vi "LSMcontroller_v66_improvedwfhandling.vi"() -> ()   [LabVIEW 2015] (continued)
                        n3642 = call "waveformsAObuffer.vi"("command"="get") -> ("AO wf out"=w516:waveform(dbl)[])  [unwired: 1 in]
                        n3643 = call "waveformsDObuffer.vi"("command"="get") -> ("DO wf out"=w513:digitalwaveform[])  [unwired: 1 in]
                        n3644 = Delete From Array(array=w516, length=1, index=w519) -> (array with subset deleted=w508:waveform(dbl)[])  [unwired: 1 out]
                        n3645 = call "correctwaveformsizetemp.vi"("new sampling frequency (Hz)"=w503, "start"=FALSE, "reference waveforms to"=w507, "Analog waveforms in"=w508, "stop"=FALSE, "Digital waveforms in"=w513) -> ("analog wf out"=w511:waveform(dbl)[], "Digital wf out"=w509:digitalwaveform[], "measpoints"=w505:i32)
                        n3646 = local write "Analog Lines Plot"(w511) -> ()
                        n3647 = call "GetNumCamFramesv2.vi"("Digital Waveform Graph"=w509) -> ("Numeric"=w510:i32)  [unwired: 10 in]
                        n3648 = local write "Digital Lines Plot"(w509) -> ()
                        n3649 = call "waveformsAObuffer.vi"("AO wf in"=w511, "command"="set") -> ()  [unwired: 1 out]
                        n3650 = call "waveformsDObuffer.vi"("DO wf in"=w509, "command"="set") -> ()  [unwired: 1 out]
                        n3651 = local read "wavdet"() -> (w506:bool)
                        n3652 = local write "Total Camera Frames"(w510) -> ()
                        n3653 = case shown="True" w506 {
                          tunnel: w505 -> [_ w522]
                          frame False {
                          }
                          frame True {
                            n3654 = local write "# of frames"(w522) -> ()
                          }
                        }
                      }
                    }
                  }
                  frame #6 {
                    w523 = FALSE ("remAO")
                    n3655 = local read "finite samples"() -> (w524:bool)
                    n3656 = local read "continuous"() -> (w525:bool)
                    n3657 = local read "wavdet"() -> (w526:bool)
                    n3658 = call "2pparameters.vi"("command"="get") -> ("params out"=w529:T10)  [unwired: 1 in]
                    n3659 = Bundle By Name(cluster=w529, "finite"=w524, "cont"=w525, "wavdet"=w526) -> (w527:T10)
                    n3660 = local write "remAO"(w523) -> ()
                    n3661 = property on="Rem AO wave" class="Bool (strict)"("Val(Sgnl)"=w523) -> ()  [unwired: 2 in, 2 out]
                    n3662 = call "2pparameters.vi"("Params in"=w527, "command"="set") -> ()  [unwired: 1 out]
                  }
                }
              }
            }
          }
          event "Add DO wave": Value Change {
            n3663 = event-data() -> ("NewVal"=w531:bool)  [unwired: 1 in, 5 out]
            n3664 = case shown="True" w531 {
              frame False {
              }
              frame True {
                n3665 = stacked-sequence {
                  seq-local: [_ _ _ _ _ w691 _ _] -> [_ _ _ _ _ _ w706 _]
                  frame #0 {
                    n3666 = local read "Measurement"() -> (w532:T4)
                    n3667 = case shown="\"X-Y-t movie\", Default" w532 {
                      frame "X-Y-t movie", Default {
                        n3668 = local read "avpp"() -> (w553:i32)
                        n3669 = local read "Angle ref"() -> (w552:dbl)
                        n3670 = local read "ROI Type"() -> (w551:u16)
                        n3671 = local read "xpixels ref"() -> (w548:i32)
                        n3672 = local read "Vx-min ref"() -> (w547:dbl)
                        n3673 = local read "Vx-max ref"() -> (w546:dbl)
                        n3674 = local read "ypixels ref"() -> (w544:i32)
                        n3675 = local read "Vy-min ref"() -> (w545:dbl)
                        n3676 = local read "Vy-max ref"() -> (w541:dbl)
                        n3677 = local read "Sampling rate"() -> (w535:dbl)
                        n3678 = local read "finite samples"() -> (w536:bool)
                        n3679 = local read "continuous"() -> (w539:bool)
                        n3680 = local read "wavdet"() -> (w540:bool)
                        n3681 = local read "# of frames"() -> (w538:i32)
                        n3682 = local read "maxbufferAI"() -> (w537:i32)
                        n3683 = local read "Override AI buffer"() -> (w533:bool)
                        n3684 = call "2pparameters.vi"("command"="get") -> ("params out"=w550:T10)  [unwired: 1 in]
                        n3685 = Bundle By Name(cluster=w550, "type"="X-Y-t movie", "avpp"=w553, "Angle Img"=w552, "Xpixels Img"=w548, "Vx-min Img"=w547, "VX-max Img"=w546, "Ypixels Img"=w544, "Vy-min Img"=w545, "Vy-max Img"=w541, "srate"=w535, "srate Img"=w535, "finite"=w536, "cont"=w539, "wavdet"=w540, "measpoints"=w538, "maxbufferAI"=w537, "Drawing Mode"=w551, "Vz-reset"=0.0, "AIoverride"=w533) -> (w542:T10)
                        n3686 = call "2pparameters.vi"("Params in"=w542, "command"="set") -> ()  [unwired: 1 out]
                      }
                      frame "X-Y-Z stack" {
                        n3687 = call "2pparameters.vi"("command"="get") -> ("params out"=w557:T10)  [unwired: 1 in]
                        n3688 = Bundle By Name(cluster=w557, "type"="X-Y-Z stack") -> (w555:T10)
                        n3689 = call "2pparameters.vi"("Params in"=w555, "command"="set") -> ()  [unwired: 1 out]
                      }
                      frame "Lifetime (scan)" {
                        n3690 = call "2pparameters.vi"("command"="get") -> ("params out"=w562:T10)  [unwired: 1 in]
                        n3691 = Bundle By Name(cluster=w562, "type"="Lifetime (scan)") -> (w560:T10)
                        n3692 = call "2pparameters.vi"("Params in"=w560, "command"="set") -> ()  [unwired: 1 out]
                      }
                      frame "Lifetime (contour)" {
                        n3693 = local read "Vy-min draw"() -> (w572:dbl)
                        n3694 = local read "Vy-max draw"() -> (w571:dbl)
                        n3695 = local read "Vx-min draw"() -> (w574:dbl)
                        n3696 = local read "Vx-max draw"() -> (w573:dbl)
                        n3697 = local read "xpixels ref"() -> (w570:i32)
                        n3698 = local read "ypixels ref"() -> (w569:i32)
                        n3699 = local read "ROI Type"() -> (w568:u16)
                        n3700 = local read "srateAODOtt"() -> (w579:dbl)
                        n3701 = local read "# of frames"() -> (w584:i32)
                        n3702 = local read "refreshtime"() -> (w576:dbl)
                        n3703 = local read "Pel"() -> (w567:dbl)
                        n3704 = local read "bin"() -> (w582:dbl)
                        n3705 = local read "Override AI buffer"() -> (w565:bool)
                        n3706 = local read "finite samples"() -> (w591:bool)
                        n3707 = local read "srateAODOtt"() -> (w578:dbl)
                        n3708 = local read "srateAODOtt"() -> (w585:dbl)
                        n3709 = local read "continuous"() -> (w590:bool)
                        n3710 = local read "Angle ref"() -> (w575:dbl)
                        n3711 = local read "wavdet"() -> (w592:bool)
                        n3712 = local read "Vx-ref"() -> (w587:dbl)
                        n3713 = local read "Vy-ref"() -> (w589:dbl)
                        n3714 = local read "avpp"() -> (w588:i32)
                        n3715 = call "tt_timeandsamples.vi"("bin"=w582, "refreshtime"=w576, "srateAODOtt"=w579, "tot#ofsamples"=w584) -> ("refreshrate"=w580:dbl, "refreshbuffer"=w581:i32, "timetracecycles"=w586:i32)  [unwired: 5 in]
                        n3716 = local read "bin"() -> (w583:dbl)
                        n3717 = call "2pparameters.vi"("command"="get") -> ("params out"=w595:T10)  [unwired: 1 in]
                        n3718 = Bundle By Name(cluster=w595, "Drawing Mode"=w568, "measpoints"=w584, "tt_cycles"=w586, "refreshbuffer"=w581, "refreshrate"=w580, "Vx-ref"=w587, "Vy-ref"=w589, "srate"=w578, "finite"=w591, "cont"=w590, "wavdet"=w592, "avpp"=w588, "srateAODO"=w585, "bufferAI"=w581, "bin"=w583, "Angle Img"=w575, "Vxminref"=w574, "Vxmaxref"=w573, "Vyminref"=w572, "Vymaxref"=w571, "Xpixels Img"=w570, "Ypixels Img"=w569, "Pel"=w567, "Vz-reset"=0.0, "AIoverride"=w565, "type"="Lifetime (contour)") -> (w593:T10)
                        n3719 = Reciprocal(x=w580) -> (1/x=w577:dbl)
                        n3720 = local write "refreshtime"(w577) -> ()
                        n3721 = call "2pparameters.vi"("Params in"=w593, "command"="set") -> ()  [unwired: 1 out]
                      }
                      frame "X-Y-Z-t movie" {
                      }
                      frame "linescan" {
                      }
                      frame "Timetrace" {
                        n3722 = local read "Vy-min draw"() -> (w605:dbl)
                        n3723 = local read "Vy-max draw"() -> (w604:dbl)
                        n3724 = local read "Vx-min draw"() -> (w607:dbl)
                        n3725 = local read "Vx-max draw"() -> (w606:dbl)
                        n3726 = local read "xpixels ref"() -> (w603:i32)
                        n3727 = local read "ypixels ref"() -> (w602:i32)
                        n3728 = local read "ROI Type"() -> (w601:u16)
                        n3729 = local read "srateAODOtt"() -> (w612:dbl)
                        n3730 = local read "# of frames"() -> (w617:i32)
                        n3731 = local read "refreshtime"() -> (w609:dbl)
                        n3732 = local read "Pel"() -> (w600:dbl)
                        n3733 = local read "bin"() -> (w615:dbl)
                        n3734 = local read "Override AI buffer"() -> (w598:bool)
                        n3735 = local read "finite samples"() -> (w624:bool)
                        n3736 = local read "srateAODOtt"() -> (w611:dbl)
                        n3737 = local read "srateAODOtt"() -> (w618:dbl)
                        n3738 = local read "continuous"() -> (w623:bool)
                        n3739 = local read "Angle ref"() -> (w608:dbl)
                        n3740 = local read "wavdet"() -> (w625:bool)
                        n3741 = local read "Vx-ref"() -> (w620:dbl)
                        n3742 = local read "Vy-ref"() -> (w622:dbl)
                        n3743 = local read "avpp"() -> (w621:i32)
                        n3744 = call "tt_timeandsamples.vi"("bin"=w615, "refreshtime"=w609, "srateAODOtt"=w612, "tot#ofsamples"=w617) -> ("refreshrate"=w613:dbl, "refreshbuffer"=w614:i32, "timetracecycles"=w619:i32)  [unwired: 5 in]
                        n3745 = local read "bin"() -> (w616:dbl)
                        n3746 = call "2pparameters.vi"("command"="get") -> ("params out"=w628:T10)  [unwired: 1 in]
                        n3747 = Bundle By Name(cluster=w628, "Drawing Mode"=w601, "measpoints"=w617, "tt_cycles"=w619, "refreshbuffer"=w614, "refreshrate"=w613, "Vx-ref"=w620, "Vy-ref"=w622, "srate"=w611, "finite"=w624, "cont"=w623, "wavdet"=w625, "avpp"=w621, "srateAODO"=w618, "bufferAI"=w614, "bin"=w616, "Angle Img"=w608, "Vxminref"=w607, "Vxmaxref"=w606, "Vyminref"=w605, "Vymaxref"=w604, "Xpixels Img"=w603, "Ypixels Img"=w602, "Pel"=w600, "Vz-reset"=0.0, "AIoverride"=w598, "type"="Timetrace") -> (w626:T10)
                        n3748 = Reciprocal(x=w613) -> (1/x=w610:dbl)
                        n3749 = local write "refreshtime"(w610) -> ()
                        n3750 = call "2pparameters.vi"("Params in"=w626, "command"="set") -> ()  [unwired: 1 out]
                      }
                      frame "Lifetime (point)" {
                      }
                    }
                  }
                  frame #1 {
                    w631 = FALSE ("wavdet")
                    n3751 = call "2pparameters.vi"("command"="get") -> ("params out"=w635:T10)  [unwired: 1 in]
                    n3752 = Bundle By Name(cluster=w635, "finite"=w631, "cont"=w631, "wavdet"=TRUE) -> (w632:T10)
                    n3753 = call "2pparameters.vi"("Params in"=w632, "command"="set") -> ()  [unwired: 1 out]
                  }
                  frame #2 {
                    n3754 = local read "DO channels"() -> (w642:u16)
                    n3755 = call "2pparameters.vi"("command"="get") -> ("params out"=w640:T10)  [unwired: 1 in]
                    n3756 = in-place {
                      in-place-border: w642 -> [w646]
                      in-place-border: [w643] -> w637
                      n3757 = in-place-cluster #51(w640) -> ("aDO"=w645:u32[])
                      n3758 = call "add channel to active arrayv2.vi"("line array in"=w645, "line to add"=w646) -> ("line array out"=w644:u32[], "addition"=w643:bool)  [unwired: 1 out]
                      n3759 = in-place-cluster #51("aDO"=w644) -> (w638:T10)
                    }
                    n3760 = local write "addDO"(w637) -> ()
                    n3761 = call "2pparameters.vi"("Params in"=w638, "command"="set") -> ()  [unwired: 1 out]
                  }
                  frame #3 {
                    n3762 = local read "addDO"() -> (w647:bool)
                    n3763 = case shown="True" w647 {
                      frame False {
                      }
                      frame True {
                        n3764 = call "Used AO lines.vi"() -> ("used AO names"=w651:string[], "used AO lines"=w653:tag[])  [unwired: 2 in]
                        n3765 = control-ref of="Analog Lines Plot"() -> (w652:refnum<vi>)
                        n3766 = control-ref of="Digital Lines Plot"() -> (w650:refnum<vi>)
                        n3767 = call "Used DO lines.vi"() -> ("used DO names"=w649:string[], "used DO lines"=w648:tag[])  [unwired: 2 in]
                        n3768 = local write "Analog Used Lines"(w653) -> ()
                        n3769 = local write "Analog Used Names"(w651) -> ()
                        n3770 = local write "Digital Used Lines"(w648) -> ()
                        n3771 = local write "Digital Used Names"(w649) -> ()
                        n3772 = call "prepDOWaveplot.vi"("DigitalGraph in"=w650, "used DO names"=w649) -> ()  [unwired: 1 in]
                        n3773 = call "prepAOWaveplot.vi"("WaveformGraph in"=w652, "Analog Used Names"=w651) -> ()  [unwired: 1 in]
                      }
                    }
                  }
                  frame #4 {
                    n3774 = local read "addDO"() -> (w654:bool)
                    n3775 = case shown="True" w654 {
                      frame False {
                      }
                      frame True {
                        n3776 = local read "Build digital waveform tabs"() -> (w655:enum32{"Simple", "Matlab"})
                        n3777 = case shown="\"Matlab\"" w655 {
                          frame "Simple", Default {
                            n3778 = local read "Meastab"() -> (w657:enum32{"X-Y Image", "Linescan", "Timetrace"})
                            n3779 = call "waveformparamsv2.vi"("command"="get") -> ("Params out"=w671:T14)  [unwired: 4 in, 2 out]
                            n3780 = case shown="\"Timetrace\"" w657 {
                              tunnel: [w673 w674] -> w656
                              frame "X-Y Image", Default {
                                n3781 = local read "Sampling rate"() -> (w673:dbl)
                              }
                              frame "Timetrace" {
                                n3782 = local read "srateAODOtt"() -> (w674:dbl)
                              }
                            }
                            n3783 = Unbundle By Name(w671) -> ("DO parameters"=w669:T17)
                            n3784 = local read "Digital padding value"() -> (w660:dbl)
                            n3785 = local read "Digital time offset (s)"() -> (w661:dbl)
                            n3786 = local read "Digital phase (s)"() -> (w663:dbl)
                            n3787 = local read "Digital Freq (Hz)"() -> (w662:dbl)
                            n3788 = local read "Digital DC (%)"() -> (w664:dbl)
                            n3789 = Index Array(array=w669, index=0) -> (element=w668:T18)
                            n3790 = Bundle By Name(cluster=w668, "Digital DC (%)"=w664, "Digital phase"=w663, "Digital Freq (Hz)"=w662, "Sampling frequency (Hz)"=w656, "Digital time offset (s)"=w661, "padding value"=w660, "matlab wave file"=path "", "DOtab"=0.0) -> (w666:T18)
                            n3791 = Build Array(w666) -> (w665:T17)
                            n3792 = call "waveformparamsv2.vi"("command"="add DO", "add DO"=w665) -> ()  [unwired: 3 in, 3 out]
                          }
                          frame "Matlab" {
                            w678 = 0.0 ("DOtab")
                            n3793 = local read "Meastab"() -> (w676:enum32{"X-Y Image", "Linescan", "Timetrace"})
                            n3794 = call "waveformparamsv2.vi"("command"="get") -> ("Params out"=w687:T14)  [unwired: 4 in, 2 out]
                            n3795 = case shown="\"Timetrace\"" w676 {
                              tunnel: [w689 w690] -> w675
                              frame "X-Y Image", Default {
                                n3796 = local read "Sampling rate"() -> (w689:dbl)
                              }
                              frame "Timetrace" {
                                n3797 = local read "srateAODOtt"() -> (w690:dbl)
                              }
                            }
                            n3798 = Unbundle By Name(w687) -> ("DO parameters"=w685:T17)
                            n3799 = local read "Matlab waveform path DO"() -> (w677:path)
                            n3800 = local read "Matlab padding value DO"() -> (w680:dbl)
                            n3801 = Index Array(array=w685, index=0) -> (element=w684:T18)
                            n3802 = Bundle By Name(cluster=w684, "Digital DC (%)"=w678, "Digital phase"=w678, "Digital Freq (Hz)"=w678, "Sampling frequency (Hz)"=w675, "Digital time offset (s)"=w678, "padding value"=w680, "matlab wave file"=w677, "DOtab"=1.0) -> (w682:T18)
                            n3803 = Build Array(w682) -> (w681:T17)
                            n3804 = call "waveformparamsv2.vi"("command"="add DO", "add DO"=w681) -> ()  [unwired: 3 in, 3 out]
                          }
                        }
                      }
                    }
                  }
                  frame #5 {
                    n3805 = local read "addDO"() -> (w692:bool)
                    n3806 = case shown="True" w692 {
                      tunnel: [_ w693] -> w691
                      frame False {
                      }
                      frame True {
                        n3807 = property on="refwf" class="Ring (strict)"() -> ("RingText.Text"=w698:string)  [unwired: 2 in, 2 out]
                        n3808 = call "waveformsDObuffer.vi"("command"="get") -> ("DO wf out"=w697:digitalwaveform[])  [unwired: 1 in]
                        n3809 = call "waveformsAObuffer.vi"("command"="get") -> ("AO wf out"=w695:waveform(dbl)[])  [unwired: 1 in]
                        n3810 = call "referfencesize.vi"("Digital waveforms in"=w697, "Analog waveforms in"=w695, "reference waveforms to"=w698) -> ("number of samples"=w693:i32)  [unwired: 2 in]
                      }
                    }
                  }
                  frame #6 {
                    n3811 = local read "Build digital waveform tabs"() -> (w709:enum32{"Simple", "Matlab"})
                    n3812 = call "waveformparamsv2.vi"("command"="get last DO") -> ("last DO"=w708:T18)  [unwired: 4 in, 2 out]
                    n3813 = local read "Meastab"() -> (w702:enum32{"X-Y Image", "Linescan", "Timetrace"})
                    n3814 = call "waveformsDObuffer.vi"("command"="get") -> ("DO wf out"=w707:digitalwaveform[])  [unwired: 1 in]
                    n3815 = case shown="\"Simple\", Default" w709 {
                      tunnel: w708 -> [w726 w728]
                      tunnel: w706 -> [w725 _]
                      tunnel: [w724 w727] -> w705
                      frame "Simple", Default {
                        n3816 = call "simple digital from wf params.vi"("waveform params"=w726, "number of samples"=w725) -> ("digital waveform"=w724:digitalwaveform)
                      }
                      frame "Matlab" {
                        n3817 = call "matlabDOwffromparam.vi"("waveform params"=w728) -> ("digital waveform"=w727:digitalwaveform)
                      }
                    }
                    n3818 = property on="refwf" class="Ring (strict)"() -> ("RingText.Text"=w712:string)  [unwired: 2 in, 2 out]
                    n3819 = case shown="\"Timetrace\"" w702 {
                      tunnel: [w721 w722] -> w701
                      frame "X-Y Image", Default {
                        n3820 = local read "Sampling rate"() -> (w721:dbl)
                      }
                      frame "Timetrace" {
                        n3821 = local read "srateAODOtt"() -> (w722:dbl)
                      }
                    }
                    n3822 = call "waveformsAObuffer.vi"("command"="get") -> ("AO wf out"=w720:waveform(dbl)[])  [unwired: 1 in]
                    n3823 = Build Array (concatenate)(w707, w705) -> (w711:digitalwaveform[])
                    n3824 = call "correctwaveformsizetemp.vi"("new sampling frequency (Hz)"=w701, "start"=FALSE, "reference waveforms to"=w712, "Analog waveforms in"=w720, "stop"=FALSE, "Digital waveforms in"=w711) -> ("analog wf out"=w715:waveform(dbl)[], "Digital wf out"=w713:digitalwaveform[], "measpoints"=w703:i32)
                    n3825 = local write "Analog Lines Plot"(w715) -> ()
                    n3826 = call "GetNumCamFramesv2.vi"("Digital Waveform Graph"=w713) -> ("Numeric"=w714:i32)  [unwired: 10 in]
                    n3827 = local write "Digital Lines Plot"(w713) -> ()
                    n3828 = call "waveformsAObuffer.vi"("AO wf in"=w715, "command"="set") -> ()  [unwired: 1 out]
                    n3829 = call "waveformsDObuffer.vi"("DO wf in"=w713, "command"="set") -> ()  [unwired: 1 out]
                    n3830 = local write "Total Camera Frames"(w714) -> ()
                    n3831 = local read "wavdet"() -> (w704:bool)
                    n3832 = case shown="True" w704 {
                      tunnel: w703 -> [_ w723]
                      frame False {
                      }
                      frame True {
                        n3833 = local write "# of frames"(w723) -> ()
                      }
                    }
                  }
                  frame #7 {
                    w730 = FALSE ("addAO")
                    n3834 = local read "Build digital waveform tabs"() -> (w729:enum32{"Simple", "Matlab"})
                    n3835 = case shown="\"Simple\", Default" w729 {
                      frame "Simple", Default {
                        n3836 = local write "not loadedDO"(FALSE ("not loadedDO")) -> ()
                      }
                      frame "Matlab" {
                        n3837 = local write "not loadedDOml"(FALSE ("not loadedDO")) -> ()
                      }
                    }
                    n3838 = local read "finite samples"() -> (w731:bool)
                    n3839 = local read "continuous"() -> (w732:bool)
                    n3840 = local read "wavdet"() -> (w733:bool)
                    n3841 = call "2pparameters.vi"("command"="get") -> ("params out"=w736:T10)  [unwired: 1 in]
                    n3842 = Bundle By Name(cluster=w736, "finite"=w731, "cont"=w732, "wavdet"=w733) -> (w734:T10)
                    n3843 = call "2pparameters.vi"("Params in"=w734, "command"="set") -> ()  [unwired: 1 out]
                    n3844 = local write "addDO"(w730) -> ()
                    n3845 = property on="Add DO wave" class="Bool (strict)"("Val(Sgnl)"=w730) -> ()  [unwired: 2 in, 2 out]
                  }
                }
              }
            }
          }
          event "DO channels": Value Change {
            n3846 = event-data() -> ()  [unwired: 1 in, 6 out]
            n3847 = local read "DO channels"() -> (w742:u16)
            n3848 = call "2pparameters.vi"("command"="get") -> ("params out"=w744:T10)  [unwired: 1 in]
            n3849 = Unbundle By Name(w744) -> ("aDO"=w743:u32[])
            n3850 = Search 1D Array(1D array=w743, element=w742) -> (index of element=w741:i32)  [unwired: 1 in]
            n3851 = Equal?(x=w741, y=-1.0) -> (x = y?=w740:bool)
            n3852 = case shown="False" w740 {
              tunnel: w741 -> [w759 _]
              frame False {
                n3853 = call "waveformparamsv2.vi"("command"="get") -> ("Params out"=w754:T14)  [unwired: 4 in, 2 out]
                n3854 = Unbundle By Name(w754) -> ("DO parameters"=w752:T17)
                n3855 = Index Array(array=w752, index=w759) -> (element=w758:T18)
                n3856 = Unbundle By Name(w758) -> ("Digital DC (%)"=w757:dbl, "Digital phase"=w756:dbl, "Digital Freq (Hz)"=w755:dbl, "Sampling frequency (Hz)"=w747:dbl, "Digital time offset (s)"=w751:dbl, "padding value"=w750:dbl, "matlab wave file"=w749:path, "DOtab"=w748:dbl)
                n3857 = local write "Build digital waveform tabs"(w748) -> ()
                n3858 = local write "Digital DC (%)"(w757) -> ()
                n3859 = local write "Matlab waveform path DO"(w749) -> ()
                n3860 = local write "Digital time offset (s)"(w751) -> ()
                n3861 = local write "Matlab padding value DO"(w750) -> ()
                n3862 = local write "Digital padding value"(w750) -> ()
                n3863 = local write "Sampling rate \ncurrent wf"(w747) -> ()
                n3864 = local write "Digital Freq (Hz)"(w755) -> ()
                n3865 = local write "Digital phase (s)"(w756) -> ()
              }
              frame True {
              }
            }
          }
          event "Rem DO wave": Value Change {
            n3866 = event-data() -> ("NewVal"=w760:bool)  [unwired: 1 in, 5 out]
            n3867 = case shown="True" w760 {
              frame False {
              }
              frame True {
                n3868 = stacked-sequence {
                  seq-local: [_ _ w866 _ _ _ _] -> [_ _ _ _ w885 w896 _]
                  frame #0 {
                    n3869 = local read "Measurement"() -> (w761:T4)
                    n3870 = case shown="\"linescan\"" w761 {
                      frame "X-Y-t movie", Default {
                        n3871 = local read "avpp"() -> (w782:i32)
                        n3872 = local read "Angle ref"() -> (w781:dbl)
                        n3873 = local read "ROI Type"() -> (w780:u16)
                        n3874 = local read "xpixels ref"() -> (w777:i32)
                        n3875 = local read "Vx-min ref"() -> (w776:dbl)
                        n3876 = local read "Vx-max ref"() -> (w775:dbl)
                        n3877 = local read "ypixels ref"() -> (w773:i32)
                        n3878 = local read "Vy-min ref"() -> (w774:dbl)
                        n3879 = local read "Vy-max ref"() -> (w770:dbl)
                        n3880 = local read "Sampling rate"() -> (w764:dbl)
                        n3881 = local read "finite samples"() -> (w765:bool)
                        n3882 = local read "continuous"() -> (w768:bool)
                        n3883 = local read "wavdet"() -> (w769:bool)
                        n3884 = local read "# of frames"() -> (w767:i32)
                        n3885 = local read "maxbufferAI"() -> (w766:i32)
                        n3886 = local read "Override AI buffer"() -> (w762:bool)
                        n3887 = call "2pparameters.vi"("command"="get") -> ("params out"=w779:T10)  [unwired: 1 in]
                        n3888 = Bundle By Name(cluster=w779, "type"="X-Y-t movie", "avpp"=w782, "Angle Img"=w781, "Xpixels Img"=w777, "Vx-min Img"=w776, "VX-max Img"=w775, "Ypixels Img"=w773, "Vy-min Img"=w774, "Vy-max Img"=w770, "srate"=w764, "srate Img"=w764, "finite"=w765, "cont"=w768, "wavdet"=w769, "measpoints"=w767, "maxbufferAI"=w766, "Drawing Mode"=w780, "Vz-reset"=0.0, "AIoverride"=w762) -> (w771:T10)
                        n3889 = call "2pparameters.vi"("Params in"=w771, "command"="set") -> ()  [unwired: 1 out]
                      }
                      frame "X-Y-Z stack" {
                        n3890 = call "2pparameters.vi"("command"="get") -> ("params out"=w786:T10)  [unwired: 1 in]
                        n3891 = Bundle By Name(cluster=w786, "type"="X-Y-Z stack") -> (w784:T10)
                        n3892 = call "2pparameters.vi"("Params in"=w784, "command"="set") -> ()  [unwired: 1 out]
                      }
                      frame "Lifetime (scan)" {
                        n3893 = call "2pparameters.vi"("command"="get") -> ("params out"=w791:T10)  [unwired: 1 in]
                        n3894 = Bundle By Name(cluster=w791, "type"="Lifetime (scan)") -> (w789:T10)
                        n3895 = call "2pparameters.vi"("Params in"=w789, "command"="set") -> ()  [unwired: 1 out]
                      }
                      frame "Lifetime (contour)" {
                        n3896 = local read "Vy-min draw"() -> (w801:dbl)
                        n3897 = local read "Vy-max draw"() -> (w800:dbl)
                        n3898 = local read "Vx-min draw"() -> (w803:dbl)
                        n3899 = local read "Vx-max draw"() -> (w802:dbl)
                        n3900 = local read "xpixels ref"() -> (w799:i32)
                        n3901 = local read "ypixels ref"() -> (w798:i32)
                        n3902 = local read "ROI Type"() -> (w797:u16)
                        n3903 = local read "srateAODOtt"() -> (w808:dbl)
                        n3904 = local read "# of frames"() -> (w813:i32)
                        n3905 = local read "refreshtime"() -> (w805:dbl)
                        n3906 = local read "Pel"() -> (w796:dbl)
                        n3907 = local read "bin"() -> (w811:dbl)
                        n3908 = local read "Override AI buffer"() -> (w794:bool)
                        n3909 = local read "finite samples"() -> (w820:bool)
                        n3910 = local read "srateAODOtt"() -> (w807:dbl)
                        n3911 = local read "srateAODOtt"() -> (w814:dbl)
                        n3912 = local read "continuous"() -> (w819:bool)
                        n3913 = local read "Angle ref"() -> (w804:dbl)
                        n3914 = local read "wavdet"() -> (w821:bool)
                        n3915 = local read "Vx-ref"() -> (w816:dbl)
                        n3916 = local read "Vy-ref"() -> (w818:dbl)
                        n3917 = local read "avpp"() -> (w817:i32)
                        n3918 = call "tt_timeandsamples.vi"("bin"=w811, "refreshtime"=w805, "srateAODOtt"=w808, "tot#ofsamples"=w813) -> ("refreshrate"=w809:dbl, "refreshbuffer"=w810:i32, "timetracecycles"=w815:i32)  [unwired: 5 in]
                        n3919 = local read "bin"() -> (w812:dbl)
                        n3920 = call "2pparameters.vi"("command"="get") -> ("params out"=w824:T10)  [unwired: 1 in]
                        n3921 = Bundle By Name(cluster=w824, "Drawing Mode"=w797, "measpoints"=w813, "tt_cycles"=w815, "refreshbuffer"=w810, "refreshrate"=w809, "Vx-ref"=w816, "Vy-ref"=w818, "srate"=w807, "finite"=w820, "cont"=w819, "wavdet"=w821, "avpp"=w817, "srateAODO"=w814, "bufferAI"=w810, "bin"=w812, "Angle Img"=w804, "Vxminref"=w803, "Vxmaxref"=w802, "Vyminref"=w801, "Vymaxref"=w800, "Xpixels Img"=w799, "Ypixels Img"=w798, "Pel"=w796, "Vz-reset"=0.0, "AIoverride"=w794, "type"="Lifetime (contour)") -> (w822:T10)
                        n3922 = Reciprocal(x=w809) -> (1/x=w806:dbl)
                        n3923 = local write "refreshtime"(w806) -> ()
                        n3924 = call "2pparameters.vi"("Params in"=w822, "command"="set") -> ()  [unwired: 1 out]
                      }
                      frame "X-Y-Z-t movie" {
                      }
                      frame "linescan" {
                      }
                      frame "Timetrace" {
                        n3925 = local read "Vy-min draw"() -> (w834:dbl)
                        n3926 = local read "Vy-max draw"() -> (w833:dbl)
                        n3927 = local read "Vx-min draw"() -> (w836:dbl)
                        n3928 = local read "Vx-max draw"() -> (w835:dbl)
                        n3929 = local read "xpixels ref"() -> (w832:i32)
                        n3930 = local read "ypixels ref"() -> (w831:i32)
                        n3931 = local read "ROI Type"() -> (w830:u16)
                        n3932 = local read "srateAODOtt"() -> (w841:dbl)
                        n3933 = local read "# of frames"() -> (w846:i32)
                        n3934 = local read "refreshtime"() -> (w838:dbl)
                        n3935 = local read "Pel"() -> (w829:dbl)
                        n3936 = local read "bin"() -> (w844:dbl)
                        n3937 = local read "Override AI buffer"() -> (w827:bool)
                        n3938 = local read "finite samples"() -> (w853:bool)
                        n3939 = local read "srateAODOtt"() -> (w840:dbl)
                        n3940 = local read "srateAODOtt"() -> (w847:dbl)
                        n3941 = local read "continuous"() -> (w852:bool)
                        n3942 = local read "Angle ref"() -> (w837:dbl)
                        n3943 = local read "wavdet"() -> (w854:bool)
                        n3944 = local read "Vx-ref"() -> (w849:dbl)
                        n3945 = local read "Vy-ref"() -> (w851:dbl)
                        n3946 = local read "avpp"() -> (w850:i32)
                        n3947 = call "tt_timeandsamples.vi"("bin"=w844, "refreshtime"=w838, "srateAODOtt"=w841, "tot#ofsamples"=w846) -> ("refreshrate"=w842:dbl, "refreshbuffer"=w843:i32, "timetracecycles"=w848:i32)  [unwired: 5 in]
                        n3948 = local read "bin"() -> (w845:dbl)
                        n3949 = call "2pparameters.vi"("command"="get") -> ("params out"=w857:T10)  [unwired: 1 in]
                        n3950 = Bundle By Name(cluster=w857, "Drawing Mode"=w830, "measpoints"=w846, "tt_cycles"=w848, "refreshbuffer"=w843, "refreshrate"=w842, "Vx-ref"=w849, "Vy-ref"=w851, "srate"=w840, "finite"=w853, "cont"=w852, "wavdet"=w854, "avpp"=w850, "srateAODO"=w847, "bufferAI"=w843, "bin"=w845, "Angle Img"=w837, "Vxminref"=w836, "Vxmaxref"=w835, "Vyminref"=w834, "Vymaxref"=w833, "Xpixels Img"=w832, "Ypixels Img"=w831, "Pel"=w829, "Vz-reset"=0.0, "AIoverride"=w827, "type"="Timetrace") -> (w855:T10)
                        n3951 = Reciprocal(x=w842) -> (1/x=w839:dbl)
                        n3952 = local write "refreshtime"(w839) -> ()
                        n3953 = call "2pparameters.vi"("Params in"=w855, "command"="set") -> ()  [unwired: 1 out]
                      }
                      frame "Lifetime (point)" {
                      }
                    }
                  }
                  frame #1 {
                    w860 = FALSE ("wavdet")
                    n3954 = call "2pparameters.vi"("command"="get") -> ("params out"=w864:T10)  [unwired: 1 in]
                    n3955 = Bundle By Name(cluster=w864, "finite"=w860, "cont"=w860, "wavdet"=TRUE) -> (w861:T10)
                    n3956 = call "2pparameters.vi"("Params in"=w861, "command"="set") -> ()  [unwired: 1 out]
                  }
                  frame #2 {
                    n3957 = local read "DO channels"() -> (w872:u16)
                    n3958 = call "2pparameters.vi"("command"="get") -> ("params out"=w870:T10)  [unwired: 1 in]
                    n3959 = in-place {
                      in-place-border: w872 -> [w877]
                      in-place-border: [w874] -> w867
                      in-place-border: [w873] -> w866
                      n3960 = in-place-cluster #52(w870) -> ("aDO"=w876:u32[])
                      n3961 = call "remove channel from active arrayv2.vi"("line array in"=w876, "line to remove"=w877) -> ("line array out"=w875:u32[], "removal"=w874:bool, "index"=w873:i32)
                      n3962 = in-place-cluster #52("aDO"=w875) -> (w868:T10)
                    }
                    n3963 = local write "remDO"(w867) -> ()
                    n3964 = call "2pparameters.vi"("Params in"=w868, "command"="set") -> ()  [unwired: 1 out]
                  }
                  frame #3 {
                    n3965 = local read "remDO"() -> (w878:bool)
                    n3966 = case shown="True" w878 {
                      frame False {
                      }
                      frame True {
                        n3967 = call "Used AO lines.vi"() -> ("used AO names"=w882:string[], "used AO lines"=w884:tag[])  [unwired: 2 in]
                        n3968 = local write "Analog Used Lines"(w884) -> ()
                        n3969 = local write "Analog Used Names"(w882) -> ()
                        n3970 = call "Used DO lines.vi"() -> ("used DO names"=w880:string[], "used DO lines"=w879:tag[])  [unwired: 2 in]
                        n3971 = control-ref of="Analog Lines Plot"() -> (w883:refnum<vi>)
                        n3972 = control-ref of="Digital Lines Plot"() -> (w881:refnum<vi>)
                        n3973 = local write "Digital Used Lines"(w879) -> ()
                        n3974 = local write "Digital Used Names"(w880) -> ()
                        n3975 = call "prepAOWaveplot.vi"("WaveformGraph in"=w883, "Analog Used Names"=w882) -> ()  [unwired: 1 in]
                        n3976 = call "prepDOWaveplot.vi"("DigitalGraph in"=w881, "used DO names"=w880) -> ()  [unwired: 1 in]
                      }
                    }
                  }
                  frame #4 {
                    n3977 = local read "remDO"() -> (w886:bool)
                    n3978 = case shown="True" w886 {
                      tunnel: w885 -> [_ w887]
                      frame False {
                      }
                      frame True {
                        n3979 = call "waveformparamsv2.vi"("command"="rem DO", "index"=w887) -> ()  [unwired: 3 in, 3 out]
                      }
                    }
                  }
                  frame #5 {
                    n3980 = local read "Meastab"() -> (w892:enum32{"X-Y Image", "Linescan", "Timetrace"})
                    n3981 = property on="refwf" class="Ring (strict)"() -> ("RingText.Text"=w899:string)  [unwired: 2 in, 2 out]
                    n3982 = call "waveformsDObuffer.vi"("command"="get") -> ("DO wf out"=w898:digitalwaveform[])  [unwired: 1 in]
                    n3983 = case shown="\"Timetrace\"" w892 {
                      tunnel: [w908 w909] -> w891
                      frame "X-Y Image", Default {
                        n3984 = local read "Sampling rate"() -> (w908:dbl)
                      }
                      frame "Timetrace" {
                        n3985 = local read "srateAODOtt"() -> (w909:dbl)
                      }
                    }
                    n3986 = call "waveformsAObuffer.vi"("command"="get") -> ("AO wf out"=w907:waveform(dbl)[])  [unwired: 1 in]
                    n3987 = Delete From Array(array=w898, length=1, index=w896) -> (array with subset deleted=w895:digitalwaveform[])  [unwired: 1 out]
                    n3988 = call "correctwaveformsizetemp.vi"("new sampling frequency (Hz)"=w891, "start"=FALSE, "reference waveforms to"=w899, "Analog waveforms in"=w907, "stop"=FALSE, "Digital waveforms in"=w895) -> ("analog wf out"=w902:waveform(dbl)[], "Digital wf out"=w900:digitalwaveform[], "measpoints"=w893:i32)
                    n3989 = local read "wavdet"() -> (w894:bool)
                    n3990 = call "waveformsAObuffer.vi"("AO wf in"=w902, "command"="set") -> ()  [unwired: 1 out]
                    n3991 = call "waveformsDObuffer.vi"("DO wf in"=w900, "command"="set") -> ()  [unwired: 1 out]
                    n3992 = local write "Analog Lines Plot"(w902) -> ()
                    n3993 = local write "Digital Lines Plot"(w900) -> ()
                    n3994 = call "GetNumCamFramesv2.vi"("Digital Waveform Graph"=w900) -> ("Numeric"=w901:i32)  [unwired: 10 in]
                    n3995 = case shown="True" w894 {
                      tunnel: w893 -> [_ w910]
                      frame False {
                      }
                      frame True {
                        n3996 = local write "# of frames"(w910) -> ()
                      }
                    }
                    n3997 = local write "Total Camera Frames"(w901) -> ()
                  }
                  frame #6 {
                    w911 = FALSE ("addAO")
                    n3998 = local read "finite samples"() -> (w912:bool)
                    n3999 = local read "continuous"() -> (w913:bool)
                    n4000 = local read "wavdet"() -> (w914:bool)
                    n4001 = local write "remDO"(w911) -> ()
                    n4002 = call "2pparameters.vi"("command"="get") -> ("params out"=w917:T10)  [unwired: 1 in]
                    n4003 = Bundle By Name(cluster=w917, "finite"=w912, "cont"=w913, "wavdet"=w914) -> (w915:T10)
                    n4004 = property on="Rem DO wave" class="Bool (strict)"("Val(Sgnl)"=w911) -> ()  [unwired: 2 in, 2 out]
                    n4005 = call "2pparameters.vi"("Params in"=w915, "command"="set") -> ()  [unwired: 1 out]
                  }
                }
              }
            }
          }
          event "load changed DO wave": Value Change {
            n4006 = event-data() -> ("NewVal"=w919:bool)  [unwired: 1 in, 5 out]
            n4007 = case shown="True" w919 {
              frame False {
              }
              frame True {
                n4008 = stacked-sequence {
                  seq-local: [_ _ w1027 _ _] -> [_ _ _ w1044 _]
                  seq-local: [_ _ w1026 _ _] -> [_ _ _ w1043 _]
                  frame #0 {
                    n4009 = local read "Measurement"() -> (w921:T4)
                    n4010 = local write "changeDO"(TRUE ("addAO")) -> ()
                    n4011 = case shown="\"X-Y-t movie\", Default" w921 {
                      frame "X-Y-t movie", Default {
                        n4012 = local read "avpp"() -> (w942:i32)
                        n4013 = local read "Angle ref"() -> (w941:dbl)
                        n4014 = local read "ROI Type"() -> (w940:u16)
                        n4015 = local read "xpixels ref"() -> (w937:i32)
                        n4016 = local read "Vx-min ref"() -> (w936:dbl)
                        n4017 = local read "Vx-max ref"() -> (w935:dbl)
                        n4018 = local read "ypixels ref"() -> (w933:i32)
                        n4019 = local read "Vy-min ref"() -> (w934:dbl)
                        n4020 = local read "Vy-max ref"() -> (w930:dbl)
                        n4021 = local read "Sampling rate"() -> (w924:dbl)
                        n4022 = local read "finite samples"() -> (w925:bool)
                        n4023 = local read "continuous"() -> (w928:bool)
                        n4024 = local read "wavdet"() -> (w929:bool)
                        n4025 = local read "# of frames"() -> (w927:i32)
                        n4026 = local read "maxbufferAI"() -> (w926:i32)
                        n4027 = local read "Override AI buffer"() -> (w922:bool)
                        n4028 = call "2pparameters.vi"("command"="get") -> ("params out"=w939:T10)  [unwired: 1 in]
                        n4029 = Bundle By Name(cluster=w939, "type"="X-Y-t movie", "avpp"=w942, "Angle Img"=w941, "Xpixels Img"=w937, "Vx-min Img"=w936, "VX-max Img"=w935, "Ypixels Img"=w933, "Vy-min Img"=w934, "Vy-max Img"=w930, "srate"=w924, "srate Img"=w924, "finite"=w925, "cont"=w928, "wavdet"=w929, "measpoints"=w927, "maxbufferAI"=w926, "Drawing Mode"=w940, "Vz-reset"=0.0, "AIoverride"=w922) -> (w931:T10)
                        n4030 = call "2pparameters.vi"("Params in"=w931, "command"="set") -> ()  [unwired: 1 out]
                      }
                      frame "X-Y-Z stack" {
                        n4031 = call "2pparameters.vi"("command"="get") -> ("params out"=w946:T10)  [unwired: 1 in]
                        n4032 = Bundle By Name(cluster=w946, "type"="X-Y-Z stack") -> (w944:T10)
                        n4033 = call "2pparameters.vi"("Params in"=w944, "command"="set") -> ()  [unwired: 1 out]
                      }
                      frame "Lifetime (scan)" {
                        n4034 = call "2pparameters.vi"("command"="get") -> ("params out"=w951:T10)  [unwired: 1 in]
                        n4035 = Bundle By Name(cluster=w951, "type"="Lifetime (scan)") -> (w949:T10)
                        n4036 = call "2pparameters.vi"("Params in"=w949, "command"="set") -> ()  [unwired: 1 out]
                      }
                      frame "Lifetime (contour)" {
                        n4037 = local read "Vy-min draw"() -> (w961:dbl)
                        n4038 = local read "Vy-max draw"() -> (w960:dbl)
                        n4039 = local read "Vx-min draw"() -> (w963:dbl)
                        n4040 = local read "Vx-max draw"() -> (w962:dbl)
                        n4041 = local read "xpixels ref"() -> (w959:i32)
                        n4042 = local read "ypixels ref"() -> (w958:i32)
                        n4043 = local read "ROI Type"() -> (w957:u16)
                        n4044 = local read "srateAODOtt"() -> (w968:dbl)
                        n4045 = local read "# of frames"() -> (w973:i32)
                        n4046 = local read "refreshtime"() -> (w965:dbl)
                        n4047 = local read "Pel"() -> (w956:dbl)
                        n4048 = local read "bin"() -> (w971:dbl)
                        n4049 = local read "Override AI buffer"() -> (w954:bool)
                        n4050 = local read "finite samples"() -> (w980:bool)
                        n4051 = local read "srateAODOtt"() -> (w967:dbl)
                        n4052 = local read "srateAODOtt"() -> (w974:dbl)
                        n4053 = local read "continuous"() -> (w979:bool)
                        n4054 = local read "Angle ref"() -> (w964:dbl)
                        n4055 = local read "wavdet"() -> (w981:bool)
                        n4056 = local read "Vx-ref"() -> (w976:dbl)
                        n4057 = local read "Vy-ref"() -> (w978:dbl)
                        n4058 = local read "avpp"() -> (w977:i32)
                        n4059 = call "tt_timeandsamples.vi"("bin"=w971, "refreshtime"=w965, "srateAODOtt"=w968, "tot#ofsamples"=w973) -> ("refreshrate"=w969:dbl, "refreshbuffer"=w970:i32, "timetracecycles"=w975:i32)  [unwired: 5 in]
                        n4060 = local read "bin"() -> (w972:dbl)
                        n4061 = call "2pparameters.vi"("command"="get") -> ("params out"=w984:T10)  [unwired: 1 in]
                        n4062 = Bundle By Name(cluster=w984, "Drawing Mode"=w957, "measpoints"=w973, "tt_cycles"=w975, "refreshbuffer"=w970, "refreshrate"=w969, "Vx-ref"=w976, "Vy-ref"=w978, "srate"=w967, "finite"=w980, "cont"=w979, "wavdet"=w981, "avpp"=w977, "srateAODO"=w974, "bufferAI"=w970, "bin"=w972, "Angle Img"=w964, "Vxminref"=w963, "Vxmaxref"=w962, "Vyminref"=w961, "Vymaxref"=w960, "Xpixels Img"=w959, "Ypixels Img"=w958, "Pel"=w956, "Vz-reset"=0.0, "AIoverride"=w954, "type"="Lifetime (contour)") -> (w982:T10)
                        n4063 = Reciprocal(x=w969) -> (1/x=w966:dbl)
                        n4064 = local write "refreshtime"(w966) -> ()
                        n4065 = call "2pparameters.vi"("Params in"=w982, "command"="set") -> ()  [unwired: 1 out]
                      }
                      frame "X-Y-Z-t movie" {
                      }
                      frame "linescan" {
                      }
                      frame "Timetrace" {
                        n4066 = local read "Vy-min draw"() -> (w994:dbl)
                        n4067 = local read "Vy-max draw"() -> (w993:dbl)
                        n4068 = local read "Vx-min draw"() -> (w996:dbl)
                        n4069 = local read "Vx-max draw"() -> (w995:dbl)
                        n4070 = local read "xpixels ref"() -> (w992:i32)
                        n4071 = local read "ypixels ref"() -> (w991:i32)
                        n4072 = local read "ROI Type"() -> (w990:u16)
                        n4073 = local read "srateAODOtt"() -> (w1001:dbl)
                        n4074 = local read "# of frames"() -> (w1006:i32)
                        n4075 = local read "refreshtime"() -> (w998:dbl)
                        n4076 = local read "Pel"() -> (w989:dbl)
                        n4077 = local read "bin"() -> (w1004:dbl)
                        n4078 = local read "Override AI buffer"() -> (w987:bool)
                        n4079 = local read "finite samples"() -> (w1013:bool)
                        n4080 = local read "srateAODOtt"() -> (w1000:dbl)
                        n4081 = local read "srateAODOtt"() -> (w1007:dbl)
                        n4082 = local read "continuous"() -> (w1012:bool)
                        n4083 = local read "Angle ref"() -> (w997:dbl)
                        n4084 = local read "wavdet"() -> (w1014:bool)
                        n4085 = local read "Vx-ref"() -> (w1009:dbl)
                        n4086 = local read "Vy-ref"() -> (w1011:dbl)
                        n4087 = local read "avpp"() -> (w1010:i32)
                        n4088 = call "tt_timeandsamples.vi"("bin"=w1004, "refreshtime"=w998, "srateAODOtt"=w1001, "tot#ofsamples"=w1006) -> ("refreshrate"=w1002:dbl, "refreshbuffer"=w1003:i32, "timetracecycles"=w1008:i32)  [unwired: 5 in]
                        n4089 = local read "bin"() -> (w1005:dbl)
                        n4090 = call "2pparameters.vi"("command"="get") -> ("params out"=w1017:T10)  [unwired: 1 in]
                        n4091 = Bundle By Name(cluster=w1017, "Drawing Mode"=w990, "measpoints"=w1006, "tt_cycles"=w1008, "refreshbuffer"=w1003, "refreshrate"=w1002, "Vx-ref"=w1009, "Vy-ref"=w1011, "srate"=w1000, "finite"=w1013, "cont"=w1012, "wavdet"=w1014, "avpp"=w1010, "srateAODO"=w1007, "bufferAI"=w1003, "bin"=w1005, "Angle Img"=w997, "Vxminref"=w996, "Vxmaxref"=w995, "Vyminref"=w994, "Vymaxref"=w993, "Xpixels Img"=w992, "Ypixels Img"=w991, "Pel"=w989, "Vz-reset"=0.0, "AIoverride"=w987, "type"="Timetrace") -> (w1015:T10)
                        n4092 = Reciprocal(x=w1002) -> (1/x=w999:dbl)
                        n4093 = local write "refreshtime"(w999) -> ()
                        n4094 = call "2pparameters.vi"("Params in"=w1015, "command"="set") -> ()  [unwired: 1 out]
                      }
                      frame "Lifetime (point)" {
                      }
                    }
                  }
                  frame #1 {
                    w1020 = FALSE ("wavdet")
                    n4095 = call "2pparameters.vi"("command"="get") -> ("params out"=w1024:T10)  [unwired: 1 in]
                    n4096 = Bundle By Name(cluster=w1024, "finite"=w1020, "cont"=w1020, "wavdet"=TRUE) -> (w1021:T10)
                    n4097 = call "2pparameters.vi"("Params in"=w1021, "command"="set") -> ()  [unwired: 1 out]
                  }
                  frame #2 {
                    n4098 = local read "DO channels"() -> (w1029:u16)
                    n4099 = call "2pparameters.vi"("command"="get") -> ("params out"=w1031:T10)  [unwired: 1 in]
                    n4100 = Unbundle By Name(w1031) -> ("aDO"=w1030:u32[])
                    n4101 = Search 1D Array(1D array=w1030, element=w1029) -> (index of element=w1027:i32)  [unwired: 1 in]
                    n4102 = Greater?(x=w1027, y=-1) -> (0:w1026:bool)
                    n4103 = case shown="True" w1026 {
                      tunnel: w1027 -> [_ w1040]
                      frame False {
                      }
                      frame True {
                        n4104 = local read "Meastab"() -> (w1034:enum32{"X-Y Image", "Linescan", "Timetrace"})
                        n4105 = local read "Digital padding value"() -> (w1035:dbl)
                        n4106 = local read "Digital time offset (s)"() -> (w1036:dbl)
                        n4107 = case shown="\"Timetrace\"" w1034 {
                          tunnel: [w1041 w1042] -> w1033
                          frame "X-Y Image", Default {
                            n4108 = local read "Sampling rate"() -> (w1041:dbl)
                          }
                          frame "Timetrace" {
                            n4109 = local read "srateAODOtt"() -> (w1042:dbl)
                          }
                        }
                        n4110 = local read "Digital Freq (Hz)"() -> (w1038:dbl)
                        n4111 = local read "Digital phase (s)"() -> (w1037:dbl)
                        n4112 = local read "Digital DC (%)"() -> (w1039:dbl)
                        n4113 = call "replace DO wf param.vi"("Digital Freq (Hz)"=w1038, "Digital DC (%)"=w1039, "Digital phase"=w1037, "Sampling frequency (Hz)"=w1033, "Digital time offset (s)"=w1036, "index of DO wave"=w1040, "padding value"=w1035) -> ()  [unwired: 4 in]
                      }
                    }
                  }
                  frame #3 {
                    n4114 = case shown="True" w1043 {
                      tunnel: w1044 -> [_ w1051]
                      frame False {
                      }
                      frame True {
                        n4115 = local read "Meastab"() -> (w1048:enum32{"X-Y Image", "Linescan", "Timetrace"})
                        n4116 = call "waveformparamsv2.vi"("command"="get") -> ("Params out"=w1067:T14)  [unwired: 4 in, 2 out]
                        n4117 = Unbundle By Name(w1067) -> ("DO parameters"=w1066:T17)
                        n4118 = property on="refwf" class="Ring (strict)"() -> ("RingText.Text"=w1073:string)  [unwired: 2 in, 2 out]
                        n4119 = case shown="\"Timetrace\"" w1048 {
                          tunnel: [w1074 w1075] -> w1047
                          frame "X-Y Image", Default {
                            n4120 = local read "Sampling rate"() -> (w1074:dbl)
                          }
                          frame "Timetrace" {
                            n4121 = local read "srateAODOtt"() -> (w1075:dbl)
                          }
                        }
                        n4122 = call "waveformsAObuffer.vi"("command"="get") -> ("AO wf out"=w1071:waveform(dbl)[])  [unwired: 1 in]
                        n4123 = call "waveformsDObuffer.vi"("command"="get") -> ("DO wf out"=w1069:digitalwaveform[])  [unwired: 1 in]
                        n4124 = call "referfencesize.vi"("Digital waveforms in"=w1069, "Analog waveforms in"=w1071, "reference waveforms to"=w1073) -> ("number of samples"=w1064:i32)  [unwired: 2 in]
                        n4125 = Index Array(array=w1066, index=w1051) -> (element=w1065:T18)
                        n4126 = call "waveformsDObuffer.vi"("command"="get") -> ("DO wf out"=w1061:digitalwaveform[])  [unwired: 1 in]
                        n4127 = call "simple digital from wf params.vi"("waveform params"=w1065, "number of samples"=w1064) -> ("digital waveform"=w1063:digitalwaveform)
                        n4128 = property on="refwf" class="Ring (strict)"() -> ("RingText.Text"=w1053:string)  [unwired: 2 in, 2 out]
                        n4129 = Replace Array Subset(array=w1061, new element=w1063, index=w1051) -> (w1052:digitalwaveform[])
                        n4130 = call "waveformsAObuffer.vi"("command"="get") -> ("AO wf out"=w1060:waveform(dbl)[])  [unwired: 1 in]
                        n4131 = local read "wavdet"() -> (w1050:bool)
                        n4132 = call "correctwaveformsizetemp.vi"("new sampling frequency (Hz)"=w1047, "start"=FALSE, "reference waveforms to"=w1053, "Analog waveforms in"=w1060, "stop"=FALSE, "Digital waveforms in"=w1052) -> ("analog wf out"=w1056:waveform(dbl)[], "Digital wf out"=w1054:digitalwaveform[], "measpoints"=w1049:i32)
                        n4133 = local write "Analog Lines Plot"(w1056) -> ()
                        n4134 = call "GetNumCamFramesv2.vi"("Digital Waveform Graph"=w1054) -> ("Numeric"=w1055:i32)  [unwired: 10 in]
                        n4135 = local write "Digital Lines Plot"(w1054) -> ()
                        n4136 = case shown="True" w1050 {
                          tunnel: w1049 -> [_ w1076]
                          frame False {
                          }
                          frame True {
                            n4137 = local write "# of frames"(w1076) -> ()
                          }
                        }
                        n4138 = call "waveformsAObuffer.vi"("AO wf in"=w1056, "command"="set") -> ()  [unwired: 1 out]
                        n4139 = call "waveformsDObuffer.vi"("DO wf in"=w1054, "command"="set") -> ()  [unwired: 1 out]
                        n4140 = local write "Total Camera Frames"(w1055) -> ()
                      }
                    }
                  }
                  frame #4 {
                    w1078 = FALSE ("addAO")
                    n4141 = local read "finite samples"() -> (w1079:bool)
                    n4142 = local read "continuous"() -> (w1080:bool)
                    n4143 = local read "wavdet"() -> (w1081:bool)
                    n4144 = local write "changeDO"(w1078) -> ()
                    n4145 = property on="load changed DO wave" class="Bool (strict)"("Val(Sgnl)"=w1078) -> ()  [unwired: 2 in, 2 out]
                    n4146 = call "2pparameters.vi"("command"="get") -> ("params out"=w1084:T10)  [unwired: 1 in]
                    n4147 = Bundle By Name(cluster=w1084, "finite"=w1079, "cont"=w1080, "wavdet"=w1081) -> (w1082:T10)
                    n4148 = local write "not loadedDO"(FALSE ("not loadedDO")) -> ()
                    n4149 = call "2pparameters.vi"("Params in"=w1082, "command"="set") -> ()  [unwired: 1 out]
                  }
                }
              }
            }
          }
          event "refwf": Value Change {
            n4150 = event-data() -> ()  [unwired: 1 in, 6 out]
            n4151 = stacked-sequence {
              frame #0 {
                n4152 = local read "Measurement"() -> (w1086:T4)
                n4153 = case shown="\"X-Y-t movie\", Default" w1086 {
                  frame "X-Y-t movie", Default {
                    n4154 = local read "avpp"() -> (w1107:i32)
                    n4155 = local read "Angle ref"() -> (w1106:dbl)
                    n4156 = local read "ROI Type"() -> (w1105:u16)
                    n4157 = local read "xpixels ref"() -> (w1102:i32)
                    n4158 = local read "Vx-min ref"() -> (w1101:dbl)
                    n4159 = local read "Vx-max ref"() -> (w1100:dbl)
                    n4160 = local read "ypixels ref"() -> (w1098:i32)
                    n4161 = local read "Vy-min ref"() -> (w1099:dbl)
                    n4162 = local read "Vy-max ref"() -> (w1095:dbl)
                    n4163 = local read "Sampling rate"() -> (w1089:dbl)
                    n4164 = local read "finite samples"() -> (w1090:bool)
                    n4165 = local read "continuous"() -> (w1093:bool)
                    n4166 = local read "wavdet"() -> (w1094:bool)
                    n4167 = local read "# of frames"() -> (w1092:i32)
                    n4168 = local read "maxbufferAI"() -> (w1091:i32)
                    n4169 = local read "Override AI buffer"() -> (w1087:bool)
                    n4170 = call "2pparameters.vi"("command"="get") -> ("params out"=w1104:T10)  [unwired: 1 in]
                    n4171 = Bundle By Name(cluster=w1104, "type"="X-Y-t movie", "avpp"=w1107, "Angle Img"=w1106, "Xpixels Img"=w1102, "Vx-min Img"=w1101, "VX-max Img"=w1100, "Ypixels Img"=w1098, "Vy-min Img"=w1099, "Vy-max Img"=w1095, "srate"=w1089, "srate Img"=w1089, "finite"=w1090, "cont"=w1093, "wavdet"=w1094, "measpoints"=w1092, "maxbufferAI"=w1091, "Drawing Mode"=w1105, "Vz-reset"=0.0, "AIoverride"=w1087) -> (w1096:T10)
                    n4172 = call "2pparameters.vi"("Params in"=w1096, "command"="set") -> ()  [unwired: 1 out]
                  }
                  frame "X-Y-Z stack" {
                    n4173 = call "2pparameters.vi"("command"="get") -> ("params out"=w1111:T10)  [unwired: 1 in]
                    n4174 = Bundle By Name(cluster=w1111, "type"="X-Y-Z stack") -> (w1109:T10)
                    n4175 = call "2pparameters.vi"("Params in"=w1109, "command"="set") -> ()  [unwired: 1 out]
                  }
                  frame "Lifetime (scan)" {
                    n4176 = call "2pparameters.vi"("command"="get") -> ("params out"=w1116:T10)  [unwired: 1 in]
                    n4177 = Bundle By Name(cluster=w1116, "type"="Lifetime (scan)") -> (w1114:T10)
                    n4178 = call "2pparameters.vi"("Params in"=w1114, "command"="set") -> ()  [unwired: 1 out]
                  }
                  frame "Lifetime (contour)" {
                    n4179 = local read "Vy-min draw"() -> (w1126:dbl)
                    n4180 = local read "Vy-max draw"() -> (w1125:dbl)
                    n4181 = local read "Vx-min draw"() -> (w1128:dbl)
                    n4182 = local read "Vx-max draw"() -> (w1127:dbl)
                    n4183 = local read "xpixels ref"() -> (w1124:i32)
                    n4184 = local read "ypixels ref"() -> (w1123:i32)
                    n4185 = local read "ROI Type"() -> (w1122:u16)
                    n4186 = local read "srateAODOtt"() -> (w1133:dbl)
                    n4187 = local read "# of frames"() -> (w1138:i32)
                    n4188 = local read "refreshtime"() -> (w1130:dbl)
                    n4189 = local read "Pel"() -> (w1121:dbl)
                    n4190 = local read "bin"() -> (w1136:dbl)
                    n4191 = local read "Override AI buffer"() -> (w1119:bool)
                    n4192 = local read "finite samples"() -> (w1145:bool)
                    n4193 = local read "srateAODOtt"() -> (w1132:dbl)
                    n4194 = local read "srateAODOtt"() -> (w1139:dbl)
                    n4195 = local read "continuous"() -> (w1144:bool)
                    n4196 = local read "Angle ref"() -> (w1129:dbl)
                    n4197 = local read "wavdet"() -> (w1146:bool)
                    n4198 = local read "Vx-ref"() -> (w1141:dbl)
                    n4199 = local read "Vy-ref"() -> (w1143:dbl)
                    n4200 = local read "avpp"() -> (w1142:i32)
                    n4201 = call "tt_timeandsamples.vi"("bin"=w1136, "refreshtime"=w1130, "srateAODOtt"=w1133, "tot#ofsamples"=w1138) -> ("refreshrate"=w1134:dbl, "refreshbuffer"=w1135:i32, "timetracecycles"=w1140:i32)  [unwired: 5 in]
                    n4202 = local read "bin"() -> (w1137:dbl)
                    n4203 = call "2pparameters.vi"("command"="get") -> ("params out"=w1149:T10)  [unwired: 1 in]
                    n4204 = Bundle By Name(cluster=w1149, "Drawing Mode"=w1122, "measpoints"=w1138, "tt_cycles"=w1140, "refreshbuffer"=w1135, "refreshrate"=w1134, "Vx-ref"=w1141, "Vy-ref"=w1143, "srate"=w1132, "finite"=w1145, "cont"=w1144, "wavdet"=w1146, "avpp"=w1142, "srateAODO"=w1139, "bufferAI"=w1135, "bin"=w1137, "Angle Img"=w1129, "Vxminref"=w1128, "Vxmaxref"=w1127, "Vyminref"=w1126, "Vymaxref"=w1125, "Xpixels Img"=w1124, "Ypixels Img"=w1123, "Pel"=w1121, "Vz-reset"=0.0, "AIoverride"=w1119, "type"="Lifetime (contour)") -> (w1147:T10)
                    n4205 = Reciprocal(x=w1134) -> (1/x=w1131:dbl)
                    n4206 = local write "refreshtime"(w1131) -> ()
                    n4207 = call "2pparameters.vi"("Params in"=w1147, "command"="set") -> ()  [unwired: 1 out]
                  }
                  frame "X-Y-Z-t movie" {
                  }
                  frame "linescan" {
                  }
                  frame "Timetrace" {
                    n4208 = local read "Vy-min draw"() -> (w1159:dbl)
